vi "Check for Ini files and create.vi"() -> ()   [LabVIEW 2023]
doc: "Check if class, property, and method files exist for current version of LabVIEW, and if not, create them. \n\nRead files into the property array action engine so data is ready for use.\n\nThis is launched asynchronously when plugin runs, so it should only happen once per LabVIEW version."
panel:
  out "(Re)Building helper files":bool
  # "Checks for BundleMagic ini files, and if they don't exist, creates them"
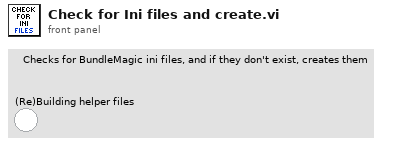
[diagram p1: front panel]
types:
  T1 = cluster{"Class Info":cluster{"Unique ID string":string, "Parent ID string":string, "Class Name (unlocalized)":string, "Class Name (localized)":string}, "Method Info":cluster{"Unique ID string":string, "Data name":string, "Short name (localized)":string, "Long name (localized)":string}, "Method Flags":cluster{"IsDeprecated":bool, "IsPrivate":bool, "IsScripting":bool, "IsNotInRun-Time":bool}, "Divider":bool}[]
  T2 = cluster{"Class":cluster{"Unique ID string":string, "Parent ID string":string, "Class Name (unlocalized)":string, "Class Name (localized)":string}, "Property":cluster{"Unique ID string":string, "Data name":string, "Short name (localized)":string, "Long name (localized)":string}, "Flags":cluster{"CanRead":bool, "CanWrite":bool, "IsDeprecated":bool, "IsPrivate":bool, "IsScripting":bool, "IsNotInRun-Time":bool, "Is Reference":bool, "Class Name":string}, "Divider":bool, "Is Write":bool, "Unwired":bool}[]
  T3 = cluster{"Class Info":cluster{"Unique ID string":string, "Parent ID string":string, "Class Name (unlocalized)":string, "Class Name (localized)":string}, "Class Heirarchy":string, "Class Type":enum16{"Unknown", "Base", "Scripting", "Private", "Deprecated", "None", "Divider"}, "Indent":u32}[]
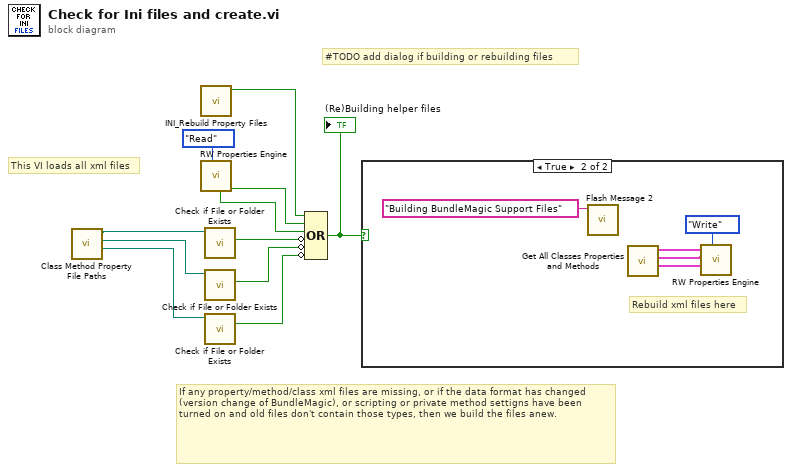
[diagram p0: block diagram]
diagram:
  # "#TODO add dialog if building or rebuilding files"
  # "If any property/method/class xml files are missing, or if the data format has changed (version change of BundleMagic), or scripting or private method settigns have been turned on and old files don't contain those types, then we build the files anew."
  # "This VI loads all xml files"
  n1 = call "Class Method Property File Paths.vi"() -> ("Method Ini"=w9:path, "Property Ini"=w10:path, "Class Ini"=w11:path)  [unwired: 8 in, 1 out]
  n2 = call "INI_Rebuild Property Files.vi"() -> ("Rebuild Property Files"=w4:bool)  [unwired: 11 in]
  n3 = call "RW Properties Engine.vi"("File Action [Read]"=enum16{"Read", "Write"}."Read") -> ("data missing?"=w3:bool, "Data format changed"=w2:bool)  [unwired: 6 in, 3 out]
  n4 = call <vilib>:"Check if File or Folder Exists.vi"("path"=w11) -> ("file or folder exists?"=w8:bool)  [unwired: 8 in, 2 out]
  n5 = call <vilib>:"Check if File or Folder Exists.vi"("path"=w10) -> ("file or folder exists?"=w7:bool)  [unwired: 8 in, 2 out]
  n6 = call <vilib>:"Check if File or Folder Exists.vi"("path"=w9) -> ("file or folder exists?"=w6:bool)  [unwired: 8 in, 2 out]
  n7 = Compound Arithmetic op=OR(w4, w3, w2, invert w8, invert w7, invert w6) -> (w5:bool)
  "(Re)Building helper files" <- w5
  n8 = case shown="True" w5 {
    frame False {
    }
    frame True {
      # "Rebuild xml files here"
      n9 = call "Flash Message 2.vi"("Dialog Message"="Building BundleMagic Support Files") -> ()  [unwired: 10 in, 1 out]
      n10 = call "Get All Classes Properties and Methods.vi"() -> ("Methods[]"=w12:T1, "Properties[]"=w13:T2, "All Classes Tree Sorted"=w14:T3)  [unwired: 8 in, 1 out]
      n11 = call "RW Properties Engine.vi"("File Action [Read]"=enum16{"Read", "Write"}."Write", "Methods[]"=w12, "Properties[]"=w13, "Classes[]"=w14) -> ()  [unwired: 3 in, 5 out]
    }
  }
